vi "Motor Control.vi"() -> ()   [LabVIEW 2012]
doc: "<B>Motor Control.vi</B> demonstrates simplistic control of a motor using PWM."
uses:
  <vilib>/Rock Robotics/SystemInterfaces/DIO/FPGA_DIORelayChannel.ctl
  <vilib>/Rock Robotics/WPI/Relay/WPI_RelayValue.ctl
  <vilib>/Rock Robotics/SystemInterfaces/Typedef/FPGA_TypedefDigitalModule.ctl
  <vilib>/Rock Robotics/WPI/Solenoid/WPI_SolenoidChannel.ctl
  <vilib>/Rock Robotics/SystemInterfaces/DIO/FPGA_DIOChannel.ctl
  StateMachineEnum.ctl
  <vilib>/Rock Robotics/WPI/Solenoid/WPI_SolenoidValue.ctl
  <vilib>/Rock Robotics/WPI/Relay/WPI_RelayDirection.ctl
  <vilib>/Rock Robotics/SystemInterfaces/DIO/FPGA_DIOPWMChannel.ctl
  <vilib>/Rock Robotics/WPI/Solenoid/WPI_SolenoidOpenSingle.vi
  <vilib>/Rock Robotics/WPI/Solenoid/WPI_SolenoidSetEnum.vi
  <vilib>/Rock Robotics/WPI/MotorControl/WPI_MotorControlOpen Talon.vi
  <vilib>/addons/control/pid/pid.llb/PID (DBL).vi
  <vilib>/Rock Robotics/WPI/Encoder/WPI_EncoderType.ctl
  <vilib>/Rock Robotics/WPI/Counter/WPI_CounterDigitalInputToDigitalSource.vi
  <vilib>/addons/control/pid/NI_PID_pid.lvlib
panel:
  in  "Pressure Switch\nand Relay Module":T1
  in  "Relay Channel":T2
  in  "Pressure Switch Channel":T3=enum."DIO 9"
  in  "Solenoid Channel":T4
  in  "Solenoid":bool
  in  "stop 2":bool
  out "Compressor Monitoring?":bool
  in  "DIO Module":T1
  in  "stop":bool
  in  "RelayValue":T5
  in  "Send Relay Off":bool
  in  "RelayChannel":T2
  out "Waveform Chart":cluster{"output":dbl, "Desired RPM":dbl}(graph)
  in  "Manual Contol?":bool=TRUE
  in  "Motor Manual":dbl(slide) step=0.01 scale=-1.0..1.0
  in  "Desired RPM":dbl step=1.0
  out "Current RPM":dbl
  in  "PID L":T6={"proportional gain (Kc)"=0.0008, "integral time (Ti, min)"=0.01, "derivative time (Td, min)"=0.0} {"derivative time (Td, min)" step=0.01 scale=0.0..0.5; "integral time (Ti, min)" step=0.01 scale=0.0..0.5; "proportional gain (Kc)" step=0.0001 scale=0.0..0.5}
  in  "Output L":cluster{"output high":dbl, "output low":dbl}={"output high"=1.0, "output low"=0.0} {"output low" step=0.1 scale=0.0..1.0; "output high" step=0.1 scale=0.0..1.0}
  in  "Stop":bool=TRUE
  out "Victor LED":bool
  # "Wiring Diagram for Digital Sidecar connected to an NI 9403"
  # "Set these inputs before running."
  # "This can be set while running."
  # "Digital Sidecar"
  # "Power\nTerminals"
  # "Motor\nTerminals"
  # "PWM cable"
  # "This shows wiring for a Victor speed controller.  The wiring is similar for a Luminary Micro Jaguar speed controller.  For a Jaguar, you must also select the appropriate instance of the Motor Open VI on the diagram."
  # "V-"
  # "M-"
  # "V+"
  # "M+"
  # "B"
  # "Innovation First"
  # "VICTOR 884"
  # "B"
  # "C"
  # "PWR"
  # "SIG"
  # "(-)"
  # "+V"
  # "10"
  # "9"
  # "8"
  # "7"
  # "6"
  # "5"
  # "4"
  # "3"
  # "2"
  # "1"
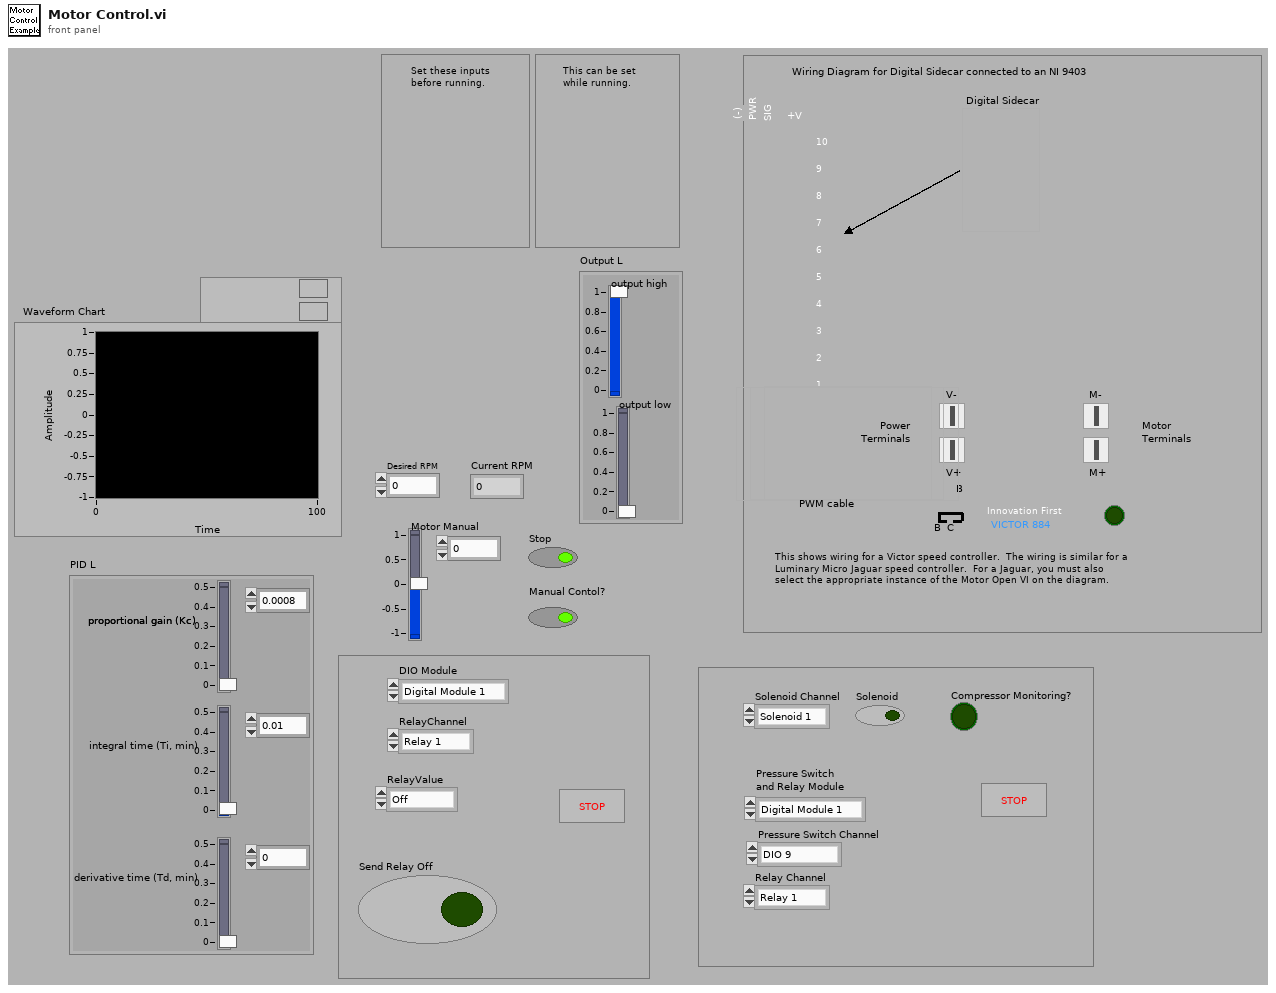
[diagram p1: front panel]
types:
  T1 = typedef "FPGA_TypedefDigitalModule.ctl" = enum16{"Digital Module 1", "Digital Module 2"}
  T2 = typedef "FPGA_DIORelayChannel.ctl" = enum8{"Relay 1", "Relay 2", "Relay 3", "Relay 4", "Relay 5", "Relay 6", "Relay 7", "Relay 8", "Invalid"}
  T3 = typedef "FPGA_DIOChannel.ctl" = enum8{"DIO 1", "DIO 2", "DIO 3", "DIO 4", "DIO 5", "DIO 6", "DIO 7", "DIO 8", "DIO 9", "DIO 10", "DIO 11", "DIO 12", "DIO 13", "DIO 14", "Invalid"}
  T4 = typedef "WPI_SolenoidChannel.ctl" = enum8{"Solenoid 1", "Solenoid 2", "Solenoid 3", "Solenoid 4", "Solenoid 5", "Solenoid 6", "Solenoid 7", "Solenoid 8", "Invalid"}
  T5 = typedef "WPI_RelayValue.ctl" = enum16{"Off", "On", "Forward", "Reverse"}
  T6 = cluster{"proportional gain (Kc)":dbl, "integral time (Ti, min)":dbl, "derivative time (Td, min)":dbl}
  T7 = typedef "StateMachineEnum.ctl" = enum16{"Init", "Idle", "Start", "Do", "Stop"}
  T8 = typedef "WPI_RelayDirection.ctl" = enum16{"Both directions", "Forward only", "Reverse only"}
  T9 = typedef "WPI_RelayDevRef.ctl" = cluster{"DevStatus":errorcluster, "Relay Channel":T2, "Digital Module":T1, "Relay Direction":T8}
  T10 = typedef "WPI_CompressorDevRef.ctl" = cluster{"DevStatus":errorcluster, "DigitalInputDevRef":T11, "RelayDevRef":T9}
  T11 = typedef "WPI_DigitalInputDevRef.ctl" = cluster{"DevStatus":errorcluster, "DIO Channel":T3, "Digital Module":T1}
  T12 = typedef "WPI_SolenoidDevRef.ctl" = cluster{"DevStatus":errorcluster, "Solenoid Module":T13, "Forward Solenoid Channel":T4, "Reverse Solenoid Channel":T4}
  T13 = typedef "FPGA_TypedefSolenoidModule.ctl" = enum16{"Solenoid Module 1", "Solenoid Module 2"}
  T14 = typedef "WPI_SolenoidValue.ctl" = enum16{"Off", "On", "Forward", "Reverse"}
  T15 = typedef "FPGA_DIOPWMChannel.ctl" = enum8{"PWM 1", "PWM 2", "PWM 3", "PWM 4", "PWM 5", "PWM 6", "PWM 7", "PWM 8", "PWM 9", "PWM 10", "Invalid"}
  T16 = typedef "WPI_EncoderType.ctl" = enum16{"1x", "2x", "4x"}
  T17 = typedef "FPGA_CounterEncoderSourceConvertionLVSourceType.ctl" = cluster{"DevStatus":errorcluster, "AnalogTriggerMode?":bool, "DigitalMode":cluster{"Digital Module":T1, "DIO Channel":T18}, "AnalogTriggerMode":cluster{"AnalogTriggerIndex":T19, "OutputType":T20}}
  T18 = typedef "FPGA_DIODigitalSourceChannel.ctl" = enum8{"DIO 1", "DIO 2", "DIO 3", "DIO 4", "DIO 5", "DIO 6", "DIO 7", "DIO 8", "DIO 9", "DIO 10", "DIO 11", "DIO 12", "DIO 13", "DIO 14", "Disabled"}
  T19 = typedef "FPGA_AnalogTriggerIndex.ctl" = enum8{"Trig 0", "Trig 1", "Trig 2", "Trig 3", "Trig 4", "Trig 5", "Trig 6", "Trig 7", "Invalid"}
  T20 = typedef "FPGA_AnalogTriggerOutType.ctl" = enum16{"InWindow", "TriggerState", "Rising", "Falling"}
  T21 = typedef "WPI_EncoderDevRef.ctl" = cluster{"DevStatus":errorcluster, "EncoderIndex":T22, "CounterIndex":T23, "DistancePerCount":dbl, "Decoding Type":T16}
  T22 = typedef "FPGA_EncoderIdx.ctl" = enum8{"Enc 0", "Enc 1", "Enc 2", "Enc 3", "Invalid"}
  T23 = typedef "FPGA_CounterCtrSystemIndex.ctl" = enum8{"Ctr 0", "Ctr 1", "Ctr 2", "Ctr 3", "Ctr 4", "Ctr 5", "Ctr 6", "Ctr 7", "Invalid"}
  T24 = typedef "WPI_MotorControlDeviceRef.ctl" = cluster{"DeviceStatus":errorcluster, "Type":enum16{"PWM", "CAN"}, "PWM":cluster{"Digital Module":T1, "PWM Channel":T15, "DeadBand":T25}, "CAN":cluster{"Device Number":u8, "Control Mode":T26, "Semaphore":T27, "Max Vout":dbl}, "Invert":bool, "TransformRef":T28, "InvTransformRef":T28}
  T25 = typedef "WPI_PWMDeadband.ctl" = cluster{"Name":string, "maxPositivePwm":i32, "minPositivePwm":i32, "centerPwm":i32, "maxNegativePwm":i32, "minNegativePwm":i32, "angularRange":u16}
  T26 = typedef "WPI_CANJaguar_ControlMode.ctl" = enum8{"Percent VBus", "Current", "Speed", "Position", "Voltage"}
  T27 = typedef "Semaphore RefNum" = refnum<k1>
  T28 = typedef "WPI_PWMTransform_ConPane.ctl" = refnum<vi>
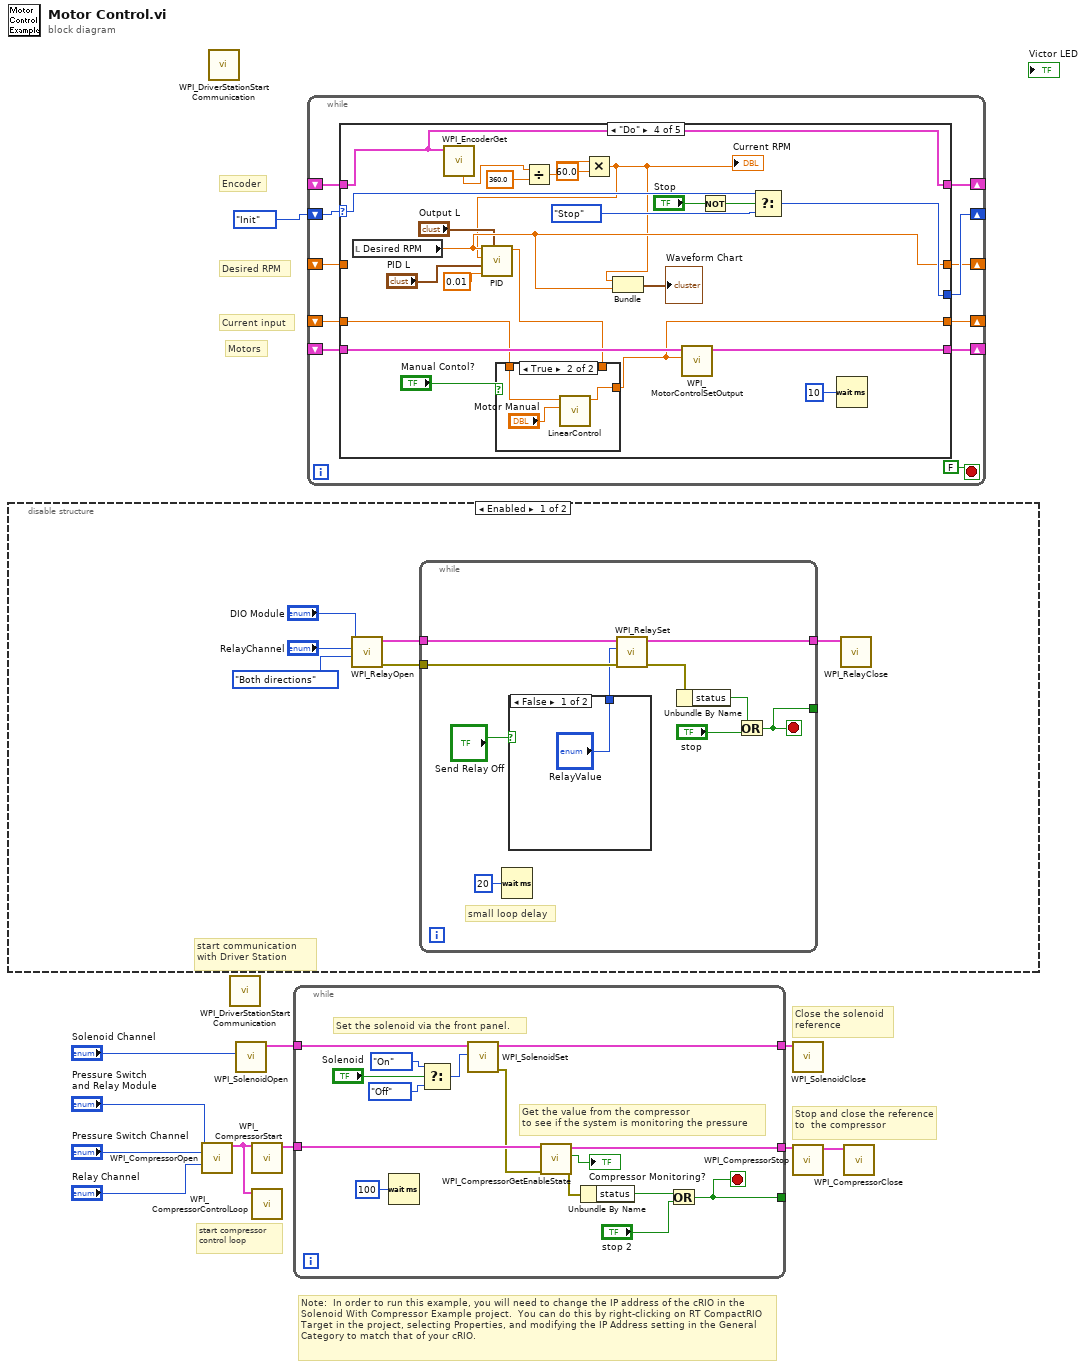
[diagram p0: block diagram]
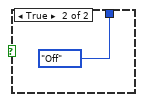
[diagram p2: hidden frame]
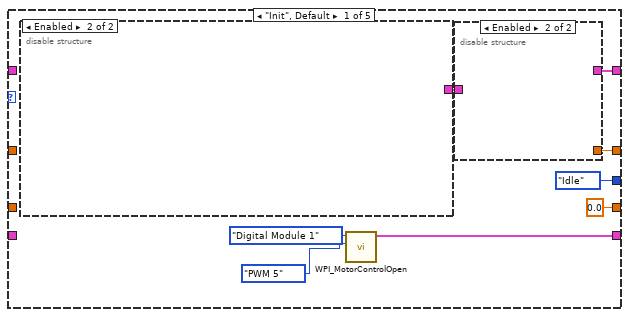
[diagram p4: hidden frame]
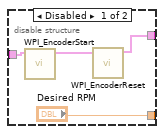
[diagram p5: hidden frame]
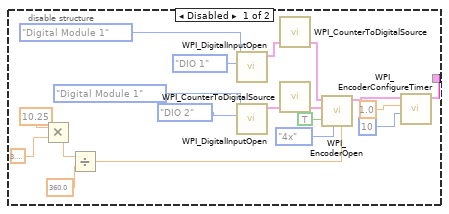
[diagram p6: hidden frame]
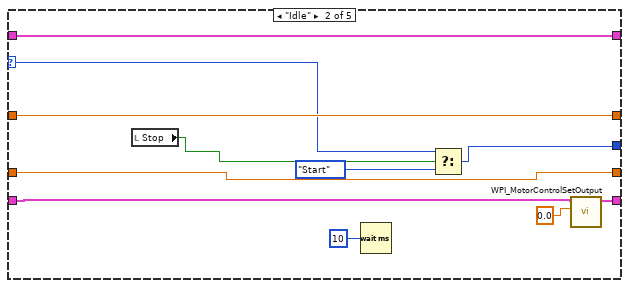
[diagram p7: hidden frame]
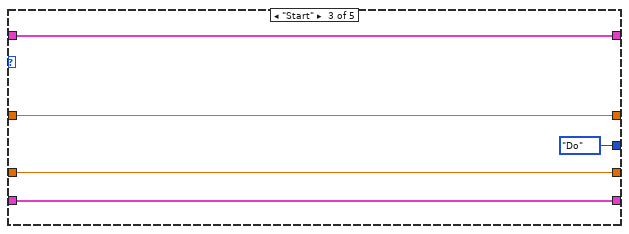
[diagram p8: hidden frame]
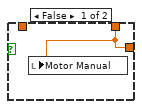
[diagram p9: hidden frame]
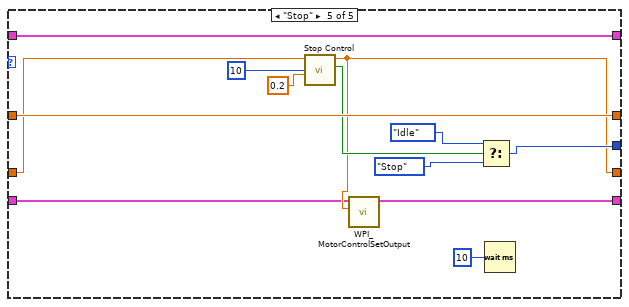
[diagram p10: hidden frame]
diagram:
  # "start compressor control loop"
  # "Note:  In order to run this example, you will need to change the IP address of the cRIO in the Solenoid With Compressor Example project.  You can do this by right-clicking on RT CompactRIO Target in the project, selecting Properties, and modifying the IP Address setting in the General Category to match that of your cRIO."
  # "Close the solenoid\nreference"
  # "Stop and close the reference to  the compressor"
  # "Current input"
  # "Desired RPM"
  # "Motors"
  # "Encoder"
  n1 = disable-structure shown="Enabled" {
    frame Enabled {
      # "start communication with Driver Station"
      n2 = call <vilib>:"WPI_RelayOpen.vi"("Relay Direction"=WPI_RelayDirection."Both directions", "Relay Channel"="RelayChannel", "Digital Module (Module 1)"="DIO Module") -> ("error out"=w12:errorcluster, "RelayDevRef"=w17:T9)  [unwired: 1 in, 6 out]
      n3 = while {
        tunnel: w17 -> [w27]
        tunnel: [w26] -> w16
        tunnel: [w21] -> _
        tunnel: w12 -> [w19]
        stop <- w21 stop-if-true
        # "small loop delay"
        n4 = Wait (ms)(milliseconds to wait=u32 20) -> ()  [unwired: 1 out]
        n5 = case shown="False" "Send Relay Off" {
          tunnel: ["RelayValue" WPI_RelayValue."Off" ("RelayValue")] -> w18
          frame False {
          }
          frame True {
          }
        }
        n6 = call <vilib>:"WPI_RelaySet.vi"("error in (no error)"=w19, "RelayValue"=w18, "RelayDevRef"=w27) -> ("error out"=w24:errorcluster, "RelayDevRef"=w26:T9)  [unwired: 7 out]
        n7 = Unbundle By Name(w24) -> ("status"=w22:bool)
        n8 = Or(x=w22, y="stop") -> (x .or. y?=w21:bool)
      }
      n9 = call <vilib>:"WPI_RelayClose.vi"("RelayDevRef"=w16) -> ()  [unwired: 1 in, 10 out]
    }
    frame Disabled {
    }
  }
  n10 = call <vilib>:"WPI_CompressorOpen.vi"("Pressure Switch Digital Module (Module 1)"="Pressure Switch\nand Relay Module", "Pressure Switch DIO Channel"="Pressure Switch Channel", "Relay Channel"="Relay Channel") -> ("CompressorDevRef"=w1:T10)  [unwired: 2 in, 10 out]
  n11 = call <vilib>:"WPI_DriverStationStart Communication.vi"() -> ()  [unwired: 1 in, 11 out]
  n12 = call <vilib>:"WPI_DriverStationStart Communication.vi"() -> ()  [unwired: 1 in, 11 out]
  n13 = call-poly <vilib>:"WPI_SolenoidOpen.vi"("Solenoid Channel"="Solenoid Channel") -> ("SolenoidDevRef"=w6:T12)  [unwired: 2 in, 8 out]
  n14 = call <vilib>:"WPI_CompressorStart.vi"("CompressorDevRef"=w1) -> ("CompressorDevRef"=w3:T10)  [unwired: 1 in, 9 out]
  n15 = call <vilib>:"WPI_CompressorControlLoop.vi"("CompressorDevRef"=w1) -> ()  [unwired: 11 in]
  n16 = while {
    tunnel: w6 -> [w44]
    tunnel: [w40] -> w5
    tunnel: w3 -> [w43]
    tunnel: [w42] -> w2
    tunnel: [w38] -> _
    stop <- w38 stop-if-true
    # "Get the value from the compressor \nto see if the system is monitoring the pressure"
    # "Set the solenoid via the front panel."
    n17 = Wait (ms)(milliseconds to wait=u32 100) -> ()  [unwired: 1 out]
    n18 = Select(t=WPI_SolenoidValue."On" ("Value"), s="Solenoid", f=WPI_SolenoidValue."Off" ("Value")) -> (s? t:f=w30:T14)
    n19 = call-poly <vilib>:"WPI_SolenoidSet.vi"("Value"=w30, "SolenoidDevRef"=w44) -> ("error out"=w39:errorcluster, "SolenoidDevRef"=w40:T12)  [unwired: 1 in, 7 out]
    n20 = call <vilib>:"WPI_CompressorGetEnableState.vi"("error in (no error)"=w39, "CompressorDevRef"=w43) -> ("error out"=w36:errorcluster, "Enabled"=→"Compressor Monitoring?":bool, "CompressorDevRef"=w42:T10)  [unwired: 7 out]
    n21 = Unbundle By Name(w36) -> ("status"=w35:bool)
    n22 = Or(x=w35, y="stop 2") -> (x .or. y?=w38:bool)
  }
  n23 = while {
    shift-right: [w51] -> _
    shift-left: StateMachineEnum."Init" -> [w54]
    shift-right: [w53] -> _
    shift-left: _ -> [w52]
    shift-right: [w50] -> _
    shift-left: _ -> [w49]
    shift-right: [w48] -> _
    shift-left: _ -> [w47]
    shift-right: [w46] -> _
    shift-left: _ -> [w45]
    stop <- FALSE stop-if-true
    n24 = case shown="\"Do\"" w54 {
      selector: w54 -> [_ w88 _ w125 _]
      tunnel: [w62 w97 w101 w123 w142] -> w53
      tunnel: w52 -> [_ w92 w101 w119 w130]
      tunnel: [StateMachineEnum."Idle" w94 StateMachineEnum."Do" w124 w132] -> w51
      tunnel: [w58 w96 w100 w121 w140] -> w50
      tunnel: w49 -> [_ w96 w100 w121 w140]
      tunnel: [w61 w95 w99 w116 w141] -> w48
      tunnel: w47 -> [_ w95 w99 _ w141]
      tunnel: [0.0 ("New Motor Input") w93 w98 w118 w131] -> w46
      tunnel: w45 -> [_ w93 w98 w117 w138]
      frame "Init", Default {
        n25 = disable-structure shown="Enabled" {
          disable-tunnel: [w68 _] -> w59
          frame Disabled {
            n26 = Multiply(x=10.25, y=3.141592653589793) -> (x*y=w72:dbl)
            n27 = Divide(x=w72, y=360.0) -> (x/y=w70:dbl)
            n28 = call <vilib>:"WPI_DigitalInputOpen.vi"("DIO Channel"=FPGA_DIOChannel."DIO 1", "Digital Module (Module 1)"=FPGA_TypedefDigitalModule."Digital Module 1") -> ("DigitalInputDevRef"=w84:T11)  [unwired: 1 in, 8 out]
            n29 = call <vilib>:"WPI_DigitalInputOpen.vi"("DIO Channel"=FPGA_DIOChannel."DIO 2", "Digital Module (Module 1)"=FPGA_TypedefDigitalModule."Digital Module 1") -> ("DigitalInputDevRef"=w85:T11)  [unwired: 1 in, 8 out]
            n30 = call-poly <vilib>:"WPI_CounterToDigitalSource.vi"("DigitalInputDevRef"=w84) -> ("Digital Source"=w83:T17)  [unwired: 6 out]
            n31 = call-poly <vilib>:"WPI_CounterToDigitalSource.vi"("DigitalInputDevRef"=w85) -> ("Digital Source"=w86:T17)  [unwired: 6 out]
            n32 = call <vilib>:"WPI_EncoderOpen.vi"("DistancePerCount"=w70, "Decoding Type"=WPI_EncoderType."4x", "Invert Direction (False)"=TRUE, "BSource"=w86, "ASource"=w83) -> ("EncoderDevRef"=w80:T21)  [unwired: 3 in, 3 out]
            n33 = call <vilib>:"WPI_EncoderConfigureTimer.vi"("Number Samples to Average"=u8 10, "Minimum Rate"=1.0, "EncoderDevRef"=w80) -> ("EncoderDevRef"=w68:T21)  [unwired: 1 in, 7 out]
          }
          frame Enabled {
          }
        }
        n34 = call-poly <vilib>:"WPI_MotorControlOpen.vi"("PWM Channel"=FPGA_DIOPWMChannel."PWM 5", "Digital Module (Module 1)"=FPGA_TypedefDigitalModule."Digital Module 1") -> ("MotorControlDeviceRef"=w62:T24)  [unwired: 8 in, 1 out]
        n35 = disable-structure shown="Enabled" {
          disable-tunnel: ["Desired RPM" _] -> w61
          disable-tunnel: w59 -> [w66 _]
          disable-tunnel: [w64 _] -> w58
          frame Disabled {
            n36 = call <vilib>:"WPI_EncoderStart.vi"("EncoderDevRef"=w66) -> ("EncoderDevRef"=w65:T21)  [unwired: 9 in, 1 out]
            n37 = call <vilib>:"WPI_EncoderReset.vi"("EncoderDevRef"=w65) -> ("EncoderDevRef"=w64:T21)  [unwired: 9 in, 1 out]
          }
          frame Enabled {
          }
        }
      }
      frame "Idle" {
        n38 = local read "Stop"() -> (w90:bool)
        n39 = Wait (ms)(milliseconds to wait=u32 10) -> ()  [unwired: 1 out]
        n40 = Select(t=w88, s=w90, f=StateMachineEnum."Start") -> (s? t:f=w94:T7)
        n41 = call <vilib>:"WPI_MotorControlSetOutput.vi"("Output"=0.0, "MotorControlDevRef"=w92) -> ("MotorControlDevRef"=w97:T24)  [unwired: 7 in, 2 out]
      }
      frame "Start" {
      }
      frame "Do" {
        n42 = local read "Desired RPM"() -> (w116:dbl)
        n43 = call <vilib>:"WPI_EncoderGet.vi"("EncoderDevRef"=w121) -> ("Rate"=w112:dbl)  [unwired: 5 in, 5 out]
        n44 = Divide(x=w112, y=360.0) -> (x/y=w110:dbl)
        n45 = Multiply(x=w110, y=60.0) -> (x*y=w103:dbl)
        "Current RPM" <- w103
        n46 = call-poly <vilib>:"PID.vi"("output range"="Output L", "dt (s)"=0.01, "PID gains"="PID L", "process variable"=w103, "setpoint"=w116) -> ("output"=w115:dbl)  [unwired: 5 in, 1 out]
        n47 = case shown="True" "Manual Contol?" {
          tunnel: [w126 w127] -> w118
          tunnel: w115 -> [w126 _]
          tunnel: w117 -> [_ w128]
          frame False {
            n48 = local write "Motor Manual"(w126) -> ()
          }
          frame True {
            n49 = call "LinearControl.vi"("Setpoint"="Motor Manual", "Motor Value"=w128) -> ("New Motor Value"=w127:dbl)  [unwired: 8 in, 1 out]
          }
        }
        n50 = Bundle(w103, "Desired RPM"=w116) -> (→"Waveform Chart":cluster{dbl, "Desired RPM":dbl})  [unwired: 1 in]
        n51 = call <vilib>:"WPI_MotorControlSetOutput.vi"("Output"=w118, "MotorControlDevRef"=w119) -> ("MotorControlDevRef"=w123:T24)  [unwired: 7 in, 2 out]
        n52 = Not(x="Stop") -> (.not. x?=w105:bool)
        n53 = Select(t=w125, s=w105, f=StateMachineEnum."Stop") -> (s? t:f=w124:T7)
        n54 = Wait (ms)(milliseconds to wait=u32 10) -> ()  [unwired: 1 out]
      }
      frame "Stop" {
        n55 = call "Stop Control.vi"("Rate (unit/s)"=0.2, "Loop Time (ms)"=u32 10, "Recieved Motor Input"=w138) -> ("Done Stopping"=w135:bool, "New Motor Input"=w131:dbl)  [unwired: 7 in]
        n56 = call <vilib>:"WPI_MotorControlSetOutput.vi"("Output"=w131, "MotorControlDevRef"=w130) -> ("MotorControlDevRef"=w142:T24)  [unwired: 7 in, 2 out]
        n57 = Select(t=StateMachineEnum."Idle" ("f"), s=w135, f=StateMachineEnum."Stop") -> (s? t:f=w132:T7)
        n58 = Wait (ms)(milliseconds to wait=u32 10) -> ()  [unwired: 1 out]
      }
    }
  }
  n59 = call <vilib>:"WPI_SolenoidClose.vi"("SolenoidDevRef"=w5) -> ()  [unwired: 1 in, 10 out]
  n60 = call <vilib>:"WPI_CompressorStop.vi"("CompressorDevRef"=w2) -> ("CompressorDevRef"=w4:T10)  [unwired: 1 in, 9 out]
  n61 = call <vilib>:"WPI_CompressorClose.vi"("CompressorDevRef"=w4) -> ()  [unwired: 1 in, 10 out]
